vi "saveImage.vi"(3 "UserDialog":bool, 4 "error in":errorcluster, 6 "bit depth":enum16{"16bits", "14bits", "12bits", "8bits"}(ring), 7 "session in":refnum<k35>, 8 "Reff ROI":T1, 9 "main ROI":T1, 10 "appended filename":string, 11 "Image in":T2) -> (0 "error out":errorcluster, 1 "numpy filename":string, 2 "png filename":string, 5 "session out":refnum<k35>)   [LabVIEW 2023]
uses:
  <vilib>/vision/Image Controls.llb/IMAQ Image.ctl
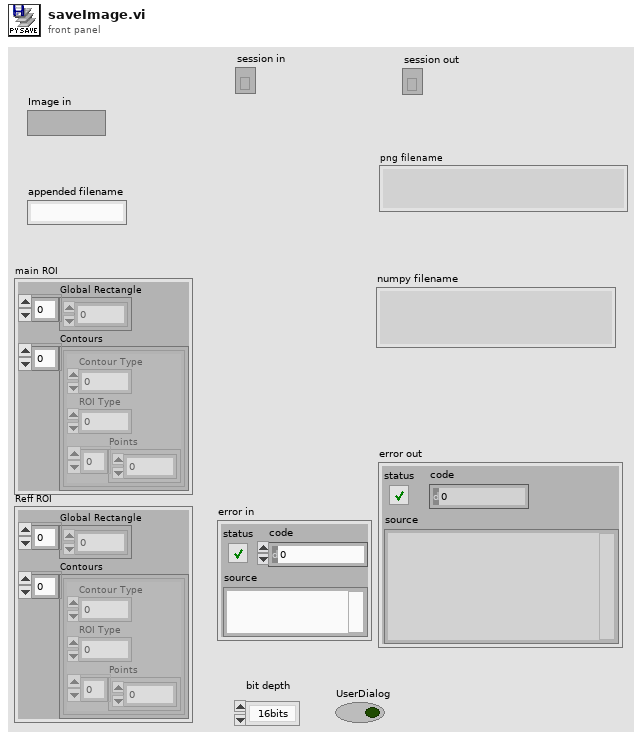
[diagram p1: front panel]
types:
  T1 = cluster{"Global Rectangle":i32[], "Contours":cluster{"Contour Type":u32, "ROI Type":u32, "Points":i32[]}[]}
  T2 = typedef "IMAQ Image.ctl" = refnum<image>
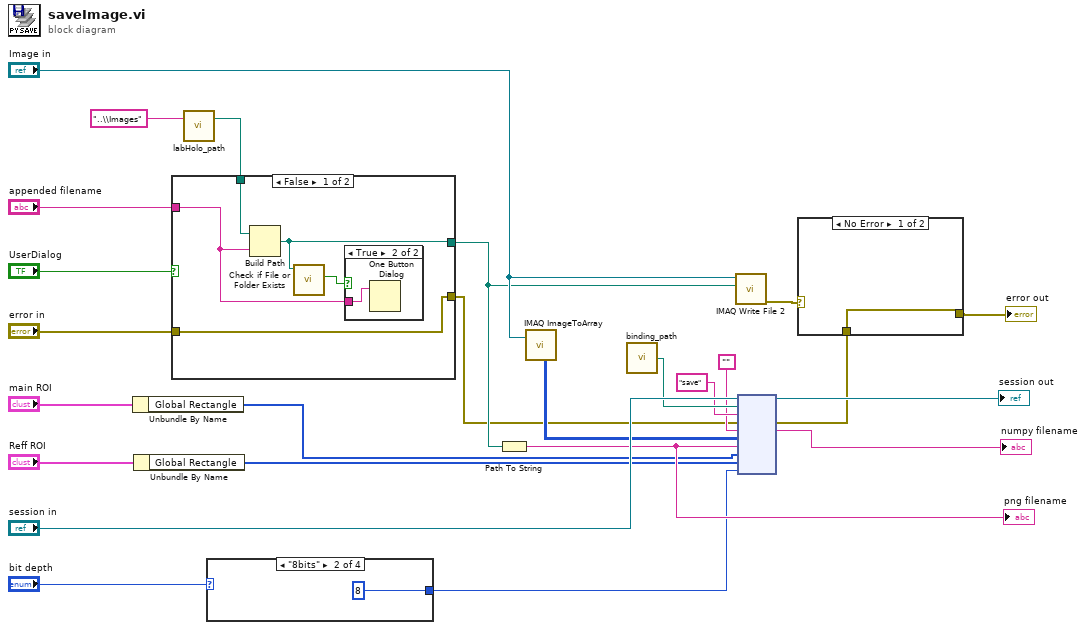
[diagram p0: block diagram]
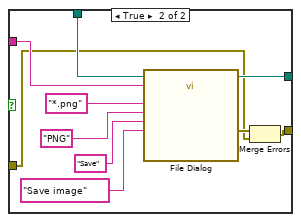
[diagram p3: hidden frame]
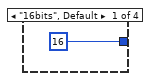
[diagram p5: hidden frame]
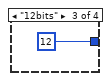
[diagram p6: hidden frame]
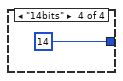
[diagram p7: hidden frame]
diagram:
  n1 = Unbundle By Name("main ROI") -> ("Global Rectangle"=w4:i32[])
  n2 = Unbundle By Name("Reff ROI") -> ("Global Rectangle"=w3:i32[])
  n3 = call "labHolo_path.vi"("sub folder or file (str)"="..\\Images") -> ("labHolo path"=w24:path)  [unwired: 1 in, 1 out]
  n4 = case shown="False" "UserDialog" {
    tunnel: "appended filename" -> [w26 w41]
    tunnel: w24 -> [w30 w40]
    tunnel: [w29 w34] -> w7
    tunnel: [w28 w35] -> w17
    tunnel: "error in" -> [w29 w32]
    frame False {
      n5 = Build Path(base path=w30, name or relative path=w26) -> (appended path=w28:path)
      n6 = call <vilib>:"Check if File or Folder Exists.vi"("path"=w28) -> ("file or folder exists?"=w27:bool)  [unwired: 8 in, 2 out]
      n7 = case shown="True" w27 {
        tunnel: w26 -> [_ w31]
        frame False {
        }
        frame True {
          n8 = One Button Dialog(message=w31) -> ()  [unwired: 1 in, 1 out]
        }
      }
    }
    frame True {
      n9 = call "File Dialog"("start path"=w40, "prompt"="Save image", "button label"="Save", "default name"=w41, "pattern (all files)"="*.png", "pattern label"="PNG") -> ("selected path"=w35:path, "error out"=w33:errorcluster)  [unwired: 6 in, 2 out]
      n10 = Merge Errors(w33, w32) -> (w34:errorcluster)
    }
  }
  n11 = case shown="\"8bits\"" "bit depth" {
    tunnel: [16 8 12 14] -> w11
    frame "16bits", Default {
    }
    frame "8bits" {
    }
    frame "12bits" {
    }
    frame "14bits" {
    }
  }
  n12 = Path To String(path=w17) -> (string=w16:string)
  "png filename" <- w16
  n13 = call "IMAQ ImageToArray"("Image"="Image in") -> ("Image Pixels (U16)"=w18:u16[][])  [unwired: 3 in, 4 out]
  n14 = call "binding_path.vi"() -> ("appended path"=w21:path)
  n15 = call-poly "IMAQ Write File 2"("File Path"=w17, "Image"="Image in") -> ("error out"=w10:errorcluster)  [unwired: 8 in, 1 out]
  n16 = node("session in", w21, "save" ("function name"), w7, "", w18, w16, w4, w3, w11) -> (→"session out":refnum<k35>, w9:errorcluster, →"numpy filename":string)  [unwired: 5 in, 2 out]
  n17 = case shown="No Error" w10 {
    selector: w10 -> [_ w47]
    tunnel: [w46 w47] -> w8
    tunnel: w9 -> [w46 _]
    frame No Error {
    }
    frame Error {
    }
  }
  "error out" <- w8
